vi "initializeStyleCollection.vi"(8 "error in (no error)":errorcluster, 11 "MS-Excel in":refnum<class "MS-Excel.lvclass">) -> (0 "error out":errorcluster, 3 "MS-Excel out":refnum<class "MS-Excel.lvclass">)   [LabVIEW 2017, in "LabVIEW NPOI.lvlib" / "MS-Excel.lvclass"]
uses:
  MS-Excel.lvclass
  MS-Excel.lvclass/MS-Excel.ctl
  Document/Document.lvclass
  C:/Users/Neo/Desktop/Dev_Tools_BR/LabVIEW_NPOI/lib/NPOI 2.1.1/NPOI.dll
  lib/NPOI 2.1.1/NPOI.dll
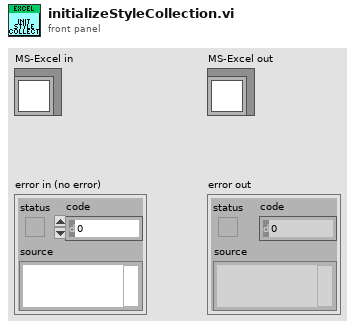
[diagram p1: front panel]
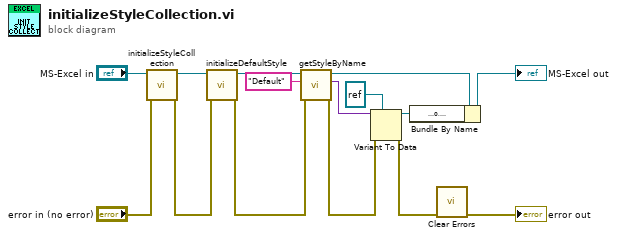
[diagram p0: block diagram]
diagram:
  n1 = call-parent "initializeStyleCollection.vi"("error in (no error)"="error in (no error)", "Document in"="MS-Excel in") -> ("error out"=w11:errorcluster, "Document out"=w13:refnum<class "MS-Excel.lvclass">)  [unwired: 8 in]
  n2 = call "initializeDefaultStyle.vi"("error in (no error)"=w11, "MS-Excel in"=w13) -> ("error out"=w9:errorcluster, "MS-Excel out"=w12:refnum<class "MS-Excel.lvclass">)  [unwired: 8 in]
  n3 = call-dynamic "getStyleByName.vi"("error in (no error)"=w9, "Style Name"="Default", "MS-Excel in"=w12) -> ("error out"=w3:errorcluster, "Style"=w6:variant, "MS-Excel out"=w10:refnum<class "MS-Excel.lvclass">)  [unwired: 6 in]
  n4 = Variant To Data(error in=w3, type=refnum<k24> refnum ("Cell Style"), Variant=w6) -> (data=w4:refnum<k24>, error out=w2:errorcluster)
  n5 = Bundle By Name(cluster=w10, "Cell Style"=w4) -> (→"MS-Excel out":refnum<class "MS-Excel.lvclass">)
  n6 = call <vilib>:"Clear Errors.vi"("error in (no error)"=w2) -> ("error out"=→"error out":errorcluster)  [unwired: 5 in, 1 out]
